vi "AlliGator All ROIs Decay Fit Non-Interactive (Fast + Individual IRF) v2.vi"(8 "error in (no error)":errorcluster, 11 "AlliGator Internal Variables DVR":refnum<data-value>) -> (0 "error out":errorcluster, 1 "Message":string, 3 "AlliGator Internal Variables DVR":refnum<data-value>)   [LabVIEW 2021, in "AlliGator Decay Fit.lvlib"]
doc: "Performs multi-ROIs NLSF decay fits for the selected ROIs.\n\nEach ROI has its own associated IRF."
uses:
  AlliGator Decay Fit.lvlib
  Internal Variables/AlliGator Internal Variables v2.ctl
  <vilib>/vision/Image Controls.llb/IMAQ Image.ctl
  Internal Variables/AlliGator Gate Image Set.ctl
  Files/AlliGator FLI Dataset Type.ctl
  Files/AlliGator Data Series Type.ctl
  Dual-Channel Datasets/AlliGator Dataset Channel.ctl
  Settings/AlliGator Gate Arithmetic.ctl
  Source Image/AlliGator Displayed Image.ctl
  Image/Named ROI Description.ctl
  Phasor Graph/AlliGator Decay Metadata v3.ctl
  Decay Preprocessing/AlliGator Decay Background Subtraction Info.ctl
  Decay Preprocessing/AlliGator Baseline Subtraction Method.ctl
  Graphs/XY Graph/XY Graph Plot Shift Parameters.ctl
  Graphs/XY Graph/XY Graph Plot Shift Method.ctl
  Decay Preprocessing/AlliGator Decay Extrapolation Parameters.ctl
  Phasor/Calibration Phasor (m, phi).ctl
  Phasor/Phasor Reference Series.ctl
  Phasor/Phasor Calibration Map v2.ctl
  Phasor/Phasor (g, s).ctl
  Phasor Graph/AlliGator Raw Phasor Plot Data v5.ctl
  Phasor/Phasor Standard Deviation Options.ctl
  Phasor Plot/AlliGator Phasor Multi-Harmonic Data.ctl
  Phasor/Phasor Harmonic Data.ctl
  Decay Fit Parameter Map/AlliGator Decay Fit Options & Parameters v3.ctl
  Fits/IRF(X)PSED/Decay Fit Options v3.ctl
  Fits/Decay Convolution/Decay Model.ctl
  Fits/Residual Type.ctl
  Fits/IRF(X)PSED/Fit Weights Type.ctl
  Fits/Non-linear Fitting Method v2.ctl
  Fits/Fit Calculation Method.ctl
  Fits/Non-linear Fitting Algorithm.ctl
  AlliGator Decay Fit Parameter Constraints 2.ctl
  Fits/IRF(X)PSED/Decay Fit Parameters In List.ctl
  Fits/IRF(X)PSED/MLE Baseline Offset Type.ctl
  Decay Preprocessing/AlliGator Decay Preprocessing Parameters.ctl
  Fits/IRF(X)PSED/Decay Fit Parameters & Derived Quantities List v2.ctl
  Fits/IRF(X)PSED/Decay Fit Result Constraint.ctl
  Decay Fit Parameter Map/AlliGator Parameter Maps Data.ctl
  Globals, Variables, Constants/AlliGator Variables List.ctl
  Settings/AlliGator Settings List.ctl
  Rich Text Box/Text Format List.ctl
  Graphs/XY Graph/XY Graph Selected Plot Info+Flag.ctl
  Graphs/XY Graph/XY Graph Refnum.ctl
  <vilib>/Utility/miscctls.llb/LVPoint32TypeDef.ctl
  Variant/Variant to Data/Variant to Boolean.vi
  Variant/Variant to Data/Variant to U16.vi
  <vilib>/Utility/error.llb/Error Cluster From Error Code.vi
  Globals, Variables, Constants/AlliGator Abort.vi
  <vilib>/ErrorRing/Error Ring.xnode
  Globals, Variables, Constants/AlliGator Globals, Variables & Constants.lvlib
  Image/Image.lvlib
  Decay Processing/AlliGator Decay Processing.lvlib
  Source Image/AlliGator Source Image.lvlib
  Strings/Strings.lvlib
  Time/Time.lvlib
  Settings/AlliGator Settings.lvlib
  Variant/Variant to Data/Variant to Data.lvlib
  GUI/GUI.lvlib
  Decay Preprocessing/AlliGator Decay Preprocessing.lvlib
  Arrays/Arrays.lvlib
  Fits/Fits.lvlib
  Notebook/Notebook.lvlib
  IRF/AlliGator IRF.lvlib
  Sound/Sound.lvlib
  Graphs/XY Graph/XY Graph Add-Ons.lvlib
  Decay Fit Parameter Map/AlliGator Decay Fit Parameter Map.lvlib
  Utilities/Utilities.lvlib
  Phasor/Phasor.lvlib
  Files/AlliGator Files.lvlib
  Internal Variables/AlliGator Internal Variables.lvlib
  Phasor Graph/AlliGator Phasor Graph.lvlib
  Phasor Plot/AlliGator Phasor Plot.lvlib
  Dual-Channel Datasets/AlliGator Dual-Channel Datasets.lvlib
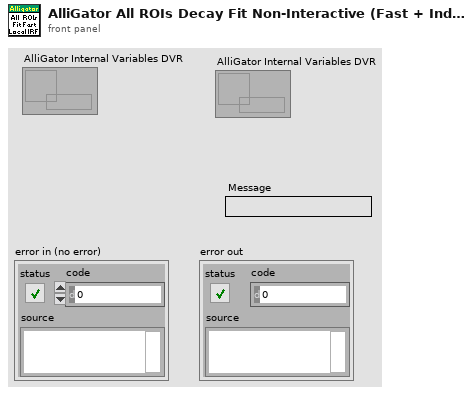
[diagram p1: front panel]
types:
  T1 = typedef "AlliGator Globals, Variables & Constants.lvlib/AlliGator Variables List.ctl" = enum16{"---- GUI ----", "GUI:Initialization Status", "GUI:State Indicators Refnum", "GUI:Original AlliGator Menu Items", "GUI:Current Action Loop State", "GUI:Script in progress", "GUI:Playback", "GUI:Loop Playback", "GUI:Search ROI Used", "GUI:Search ROI", "Decay Graph Max Legend Size", "Intensity Graph Max Legend Size", "Decay Statistics Graph Max Legend Size", "Phasor Graph Max Legend Size", "Phasor Ratio Graph Max Legend Size", "Lifetime Graph Max Legend Size", "---- Files ----", "Files:Export Dataset Frames as Individual Files", "Files:Show Batch Export Help Balloons", "Files:Frames in Dataset", "Files:ptu File Frame Start Indices", "Files:Current Frame in Dataset", "Files:Current Frame Timestamp", "Files:Dataset Loaded", "Files:Dataset Metadata", "Files:Dataset Channel", "Files:Dataset Data Description", "Files:Background Dataset Metadata", "Files:Background Dataset Channel", "Files:Background Dataset Data Description", "Files:Background File Subtraction", "Files:Background File Path", "Files:Background File Pile-up Correction", "Files:Background File Pixel Well Capacity", "Files:Background File Scaling Factor", "Files:Current Dataset Load Settings", "Files:Dataset Path", "Files:ICCD-specific Information", "Files:Macrotime Gate Separation", "------ Python Plugins ------", "Python Plugins:Information", "Python Plugins:Python Session", "Python Plugins:Valid Python Session?", "---- Source Image ----", "Source Image:ROIs", "Source Image:Current ROI", "Source Image:ROI Event Refnum", "X_Source Image:Display Range", "X_Source Image:Palette Information", "X_Source Image:Type of Displayed Image", "X_Time Gate Slider", "Source Image:Palette List", "Source Image:Scale", "Source Image:ROI Overlay Color", "Source Image:Overlay to Erase", "Source Image:Is Displayed Image Accumulated", "Source Image:White Light Image Modified", "Source Image:Mask Image Modified", "---- Image Profile Window ----", "Image Profile:Window Event Refnum", "Image Profile:IntensityType", "Image Profile:Intensity Average Type", "Image Profile:Intensity-weighted SDV", "Image Profile:Box Profile Type", "Image Profile:Window Open", "Image Profile:Plotted Fit Parameter", "------ Phasor Graph -------", "Phasor Graph:Show Line", "---- Phasor Plot ---", "Phasor Plot:Parameters Changed", "Phasor Plot:FLI Dataset Modified since last Calculation", "Phasor Harmonics Data", "Selected Phasor Harmonics", "Phasor Harmonic Manager Event Refnum", "Phasor Plot:ROIs", "Phasor Plot:Current ROI", "Phasor Plot:ROI Event Refnum", "Phasor Plot:Image Reference Points", "Phasor Plot:Computed", "Phasor Plot:Palette Information", "Phasor Plot:Palette List", "Phasor Plot:Phasor Ratio Palette Information", "Phasor Plot:Phasor Ratio Palette List", "Phasor Plot:Image Scale", "Phasor Plot:Image Overlay to Erase", "Phasor Plot:Image Elements to Update", "Phasor Plot:Current Calculation Parameters", "Phasor Plot:Current Calibration Options", "Phasor Plot:Reset Cumulated Phasor Plot", "Phasor Plot:Reference 1", "Phasor Plot:Lifetime Reference 1", "Phasor Plot:Reference 1 Frequency", "Phasor Plot:Reference 2", "Phasor Plot:Lifetime Reference 2", "Phasor Plot:Reference 2 Frequency", "---- Decay Analysis ----", "Number of Selected Decays to Fit", "LS Fit Results", "LAR Fit Results", "BS Fit Results", "Last Decay Max - Min", "Best Fit Parameters", "Best Fit Parameter Names", "Actual Size X", "Actual Size Y", "Binning X", "Binning Y", "Actual # Gates", "Dataset Number", "Gates to...", "Gates Skipped", "Gates to keep", "Gate Step", "Gate Separation", "Reversed Gates", "Pile-up Correction", "Pixel Well Capacity", "Background Subtracted", "Background Subtraction Method", "Background Definition Range", "Background File (deprecated)", "Number of Dataset Accumulated", "Array of Accumulated Dataset Paths", "Do Averaged Datasets", "Destination File Path", "Process Plot Target", "Use 1/D as Phasor Frequency", "---- Decay Fit Parameter Map -----", "Decay Fit Parameter Map:Palette Information", "Decay Fit Parameter Map:Palette List", "Decay Fit Parameter Map:X Resolution", "Decay Fit Parameter Map:Y Resolution", "Decay Fit Parameter Map:Use Decay Fit Result Constraints", "Decay Fit Parameter Map:Decay Fit Result Constraints", "Decay Fit Parameter Map:Decay Fit Result Constraints Applied", "---- Parameter Map ----", "Parameter Map:Palette Information", "Parameter Map:Palette List", "------- Local Decay Window ---------", "Local Decay Graph Window:Event Refnum", "Local Decay Graph Window:Use normalized IRF for convolution", "----- Miscellaneous ----", "Misc:Skippable Dialog Windows Status"}
  T2 = typedef "IMAQ Image.ctl" = refnum<image>
  T3 = typedef "AlliGator Settings.lvlib/AlliGator Settings List.ctl" = enum16{"GUI:Visible Settings Tab", "GUI:Last Run Version", "Source Image:Use Image Histogram for Contrast", "Source Image:Low Count Pixels Rejection Options", "Source Image:High Count Pixels Rejection Options", "Source Image:Use Image Brightness", "Source Image:Blend Overlay with Image Background", "Source Image:Use Fixed ROI Diameter", "Source Image:ROI Diameter", "Source Image:ROI Center Color", "Source Image:Peak Threshold", "Source Image:Intensity Threshold", "Source Image:Image Binning Options", "Source Image:Image Smoothing Options", "Source Image:Image Histogram Active", "Source Image:Invert Binary Mask", "Source Image:Hot Pixel Removal", "Source Image:Overlay Analyzed ROI Center", "Source Image:Auto-Adjust Contrast", "Source Image:Histogram Lower Percentile", "Source Image:Histogram Upper Percentile", "Source Image:Save Source Image", "Source Image:Scale Bar Options", "Source Image:Image Resolution (Pixel Size)", "Source Image:Flatfield Correction", "Source Image:Show Dead Left Columns Correction", "Source Image:Dead Left Columns Correction", "Source Image:Image Pre-Processing Operations Order", "Source Image:Overlay ROI Median", "Source Image:Median Overlay Color", "Data Information:Gate Width", "Data Information:Nanotime Gate Separation", "Data Information:Macrotime Gate Separation", "Data Information:Gate Step", "Data Information:# Gates", "Data Information:Gate Image Exposure", "Data Information:Gate Image Integration", "Data Information:Gates to Skip", "Data Information:Gates to Keep", "Data Information:Define Gates to", "Data Information:Channel Name", "Data Information:Available Channel Names", "Data Information:Channel Arithmetic", "Data Information:Background File Subtraction", "Data Information:Background File", "Data Information:Background Scaling Factor", "Data Information:Background Pile-up Correction", "Data Information:Background Pixel Well Capacity", "Data Information:Laser Period", "Data Information:SYNC Period", "Data Information:Pile-up Correction", "Data Information:Pixel Well Capacity", "Data Information:Dataset Scaling Factor", "Fluorescence Decay_Decay Pre-Processing:Reverse Gates", "Fluorescence Decay_Decay Pre-Processing:Verbose Decay Pre-Processing", "Fluorescence Decay_Decay Pre-Processing:Use Decay Pre-Processing", "Fluorescence Decay_Decay Pre-Processing:Background Subtraction", "Fluorescence Decay_Decay Pre-Processing:Background Definition Range", "Fluorescence Decay_Decay Pre-Processing:Baseline Subtraction Method", "Fluorescence Decay_Decay Pre-Processing:Decay Pre-Processing Operations Order", "Fluorescence Decay_Decay Pre-Processing:Smoothing Parameter", "Fluorescence Decay_Decay Pre-Processing:Shift Decay", "Fluorescence Decay_Decay Pre-Processing:Decay Shift Parameters", "Fluorescence Decay_Decay Pre-Processing:Fold Decay", "Fluorescence Decay_Decay Pre-Processing:# Folds", "Fluorescence Decay_Decay Pre-Processing:1-Normalize Decay", "Fluorescence Decay_Decay Pre-Processing:[0-1]-Normalize Decay", "Fluorescence Decay_Decay Pre-Processing:Smoothen Decay", "Fluorescence Decay_Decay Pre-Processing:Extrapolate Decay", "Fluorescence Decay_Decay Pre-Processing:Use Periodicity", "Fluorescence Decay_Decay Pre-Processing:Use Cursors", "Fluorescence Decay_Decay Pre-Processing:Tail Fraction", "Fluorescence Decay_Decay Pre-Processing:Head Fraction", "Fluorescence Decay_Decay Pre-Processing:Additional Points", "Fluorescence Decay_Decay Pre-Processing:Straighten Decay", "Fluorescence Decay_Decay Pre-Processing:Constant Background", "Fluorescence Decay_Decay Pre-Processing:Pixel-Normalize Decay", "Fluorescence Decay_Advanced Analysis:Extract IRF instead of Decay", "Fluorescence Decay_Advanced Analysis:IRF Extraction Options", "Fluorescence Decay_Advanced Analysis:IRF Optimization Options", "Fluorescence Decay_Advanced Analysis:Square Pulse Options", "Fluorescence Decay_Advanced Analysis:IRF Order", "Fluorescence Decay_Advanced Analysis:IRF Time Constants", "Fluorescence Decay_Advanced Analysis:Wavelet Analysis Options", "Fluorescence Decay_Advanced Analysis:Average Lifetime Options", "Fluorescence Decay_Fit Options:Fit Options", "Fluorescence Decay_Fit Options:Use Legacy Fitting Approach", "Fluorescence Decay_Fit Options:Use Data Information Laser Period", "Fluorescence Decay_Fit Parameters:Displayed Fit Parameters", "Fluorescence Decay_Fit Parameters:Fit Parameter Constraints", "Fluorescence Decay_Fit Parameters:Export Tabulated Results", "Fluorescence Decay_Fit Parameters:MLE Baseline Offset Type", "Fluorescence Decay_Fit Parameters:MLE Baseline Offset", "Fluorescence Decay_Fit Parameters:Guess Parameter Names", "Fluorescence Decay_Fit Parameters:Guess Parameter Values", "Fluorescence Decay_Fit Parameters:Guess Parameters Options", "Fluorescence Decay_Fit Parameters:Optimal Offset Selection Criterion", "Fluorescence Decay_Styles:Show Last Decay Only", "Fluorescence Decay_Styles:Decay Graph Color Array", "Fluorescence Decay:Decay Graph Active", "Fluorescence Decay Statistics:Min Peak Value", "Fluorescence Decay Statistics:Reject Low Decay Peak Pixels", "Fluorescence Decay Statistics:Reject High Decay Peak Pixels", "Fluorescence Decay Statistics:Max Peak Value", "Time Traces:Use File Timestamp", "Time Traces:Time Step", "Time Traces:Use Intensity Correction File", "Time Traces:Intensity Correction File", "Phasor Plot:Phasor Plot Smoothing Options", "Phasor Plot:Phasor Plot Size", "Phasor Plot:Phasor Plot Graphics Options", "Phasor Plot:Cumulative Phasor Plot", "Phasor Plot:Use Phasor Brightness", "Phasor Plot:Blend Overlay with Phasor Background", "Phasor Plot:Save Phasor Plot", "Phasor Plot:Show References", "Phasor Plot:Phasor Ratio Decay Range", "Phasor Plot:Exponential Fading", "Phasor Plot:Phasor Ratio Reference Colors", "Phasor Plot:Reference Radius", "Phasor Plot:Show Color Map Vertices", "Phasor Plot:Phasor Plot Active", "Phasor Plot:Phasor Ratio Color Map Type", "Phasor Plot:Phasor Ratio Color Map", "Phasor Plot:Phasor Ratio Display Range", "Phasor Plot:Selected Image ROI(s)", "Phasor Plot:All Image ROIs", "Phasor Plot:Selected Phasor Plot ROI(s)", "Phasor Plot:All Phasor Plot ROIs", "Phasor Plot:Phasor Ratio Color-Coded Quantity", "Phasor Plot:Store Phasor Harmonics", "Phasor Plot:Draw Reference Segment", "Phasor Plot:User-Defined Quantity", "Phasor Plot:Color Scale High Color", "Phasor Plot:Color Scale Low Color", "Phasor Plot:Intensity-weighted Phasor Plot", "Phasor Graph:Phasor Frequency", "Phasor Graph:Phasor Ratio Type", "Phasor Graph:Pixel-level Phasor Computation", "Phasor Graph:Save Phasor Graph", "Phasor Graph:Phasor Graph Active", "Phasor Graph:Phasor SDV Options", "Phasor Graph:Intensity-weighted Phasor Graph", "Phasor Graph:Define Shortest Lifetime as", "Phasor Calibration:Use Backup Calibration if needed", "Phasor Calibration:Backup Calibration Type", "Phasor Calibration:Calibration Type", "Phasor Calibration:Calibration Lifetime", "Phasor Calibration:Calibration Map Algorithm", "Single-Exponential Phasor Locus (SEPL):Gate Parameters", "Single-Exponential Phasor Locus (SEPL):User-defined Gate", "Single-Exponential Phasor Locus (SEPL):User-defined IRF", "Single-Exponential Phasor Locus (SEPL):Phasor Parameters", "Single-Exponential Phasor Locus (SEPL):Decay & IRF Parameters", "Single-Exponential Phasor Locus (SEPL):Display Parameters", "Lifetime Analysis:Decay Analysis Parameters", "Lifetime Analysis:Lifetime Map Active", "Plugins:Python Settings", "Miscellaneous:Verbose Mode", "Miscellaneous:Beep after Script", "Miscellaneous:Saved Image File Format", "Miscellaneous:Exported Gate Image Settings", "Miscellaneous:Include Loading in Timing", "Miscellaneous:Verbose Settings Mode", "Miscellaneous:Histogram Options", "Miscellaneous:Beep on Error", "Miscellaneous:# Logical Processors Used", "Miscellaneous:ROI Description Max Characters", "Miscellaneous:Verbose Error Mode", "Miscellaneous:Transparent Mask Color"}
  T4 = typedef "Image.lvlib/Named ROI Description.ctl" = cluster{"ROI Descriptor":T5, "ROI Name":string, "Overlay Color":u32}
  T5 = typedef "ROI Descriptor" = cluster{"Global Rectangle":i32[], "Contours":cluster{"ID":enum32{"External", "Internal"}, "Type":u32, "Coordinates":i32[]}[]}
  T6 = typedef "Notebook.lvlib/Text Format List.ctl" = enum16{"Message", "Result", "Error", "Setting", "Verbose", "Warning"}
  T7 = typedef "AlliGator Internal Variables.lvlib/AlliGator Internal Variables v2.ctl" = cluster{"----------------------------- Images -----------------------------":u8, "Displayed Image":T2, "White Light Image":T2, "Mask Image":T2, "ROI Mask Image":T2, "Current Dataset Images 1":T8, "Background Dataset Images 1":T8, "Current Dataset Images 2":T8, "Background Dataset Images 2":T8, "Current Dataset Arithmetic Images":T8, "Accumulated Dataset Images 1":T8, "Accumulated Dataset Images 2":T8, "Accumulated Dataset Arithmetic Images":T8, "----------------------------- File Paths -----------------------------":u8, "Phasor Plot Image":T2, "Decay Fit Parameter Map Image":T2, "Parameter Map Image":T2, "Single Data Point Path":path, "White Light Image Path":path, "Mask Image Path":path, "Time-Series Folder":path, "[Time-Series Paths]":path[], "----------------------------- FLI Dataset -----------------------------":u8, "Current Dataset":i32, "Single Dataset Type":T9, "Current Folder":string, "AlliGator Data Series Type":T10, "# Datasets":i32, "Dual-Channel Dataset":bool, "Selected Channel Name":string, "Dataset Channel":T11, "Channel Arithmetic":T12, "Dual-Channel Background Dataset":bool, "Background Channel":T11, "Dual-Channel Accumulated Dataset":bool, "Start Time":dbl, "[Time-Series Timestamps]":dbl[], "[Intensity Corrections]":dbl[], "Time Series Script":bool, "Type of Displayed Image":T13, "Gate Image Slide":u16, "# Gates":i32, "ROIs":T4[], "----------------------------- Decays -----------------------------":u8, "ROI Decay":cluster{"t Array":dbl[], "I Array":dbl[]}, "Valid Decay":bool, "Decay  Metadata":T14, "Reference Decay Plot Name":string, "Reference Decay":cluster{"t Array":dbl[], "I Array":dbl[]}, "Decay Shift Plot":cluster{"Time Stamps":dbl[], "Decay Shifts":dbl[]}, "[Decays Max Values]":sgl[], "[Decays Min Values]":sgl[], "----------------------------- Calibration -----------------------------":u8, "Calibration Phasor":T20, "Calibration Phasor Series":T21, "Phasor Calibration Map":T22, "Calibration Map MD5 Digest":string, "----------------------------- Phasor Graph -----------------------------":u8, "Last Raw Phasor":T23, "Last Calibrated Phasor":T23, "Last Calibrated Phasor SDV":T23, "Phasor Graph:Phasor Plot":cluster{"g Array":dbl[], "s Array":dbl[]}, "Phasor Graph:Phasor SDV Plot":cluster{"g Array":dbl[], "s Array":dbl[]}, "[Phasor Graph:Raw Phasor Plots]":T24[], "Phasor Plot locked to Ref 1":i32, "[Phasor Plot(s) locked to Ref 1]":i32[], "[Phasor Plot(s) locked to Ref 2]":i32[], "[Pixel Phasors]":T23[], "----------------------------- Phasor Plot -----------------------------":u8, "[[Sum Image]]":dbl[][], "[[CSG Phasors]]":csg[][], "[[Valid Pixel?]]":bool[][], "[[Phasor Ratios]]":dbl[][], "[[Average Lifetimes]]":dbl[][], "Amplitude Weighted Average Lifetime":bool, "I/m/phi Dataset":cluster{"I/m/phi Dataset?":bool, "Base Frequency":dbl[unit], "Harmonic Orders":u8[]}, "Multi Phasor Plot Data":T26, "----------------------------- Decay Fit Parameter Map -----------------------------":u8, "Decay Fit Options & Parameters":T28, "Fit Options: Decay Preprocessing Parameters":T39, "Fit Options: Reference Decay":cluster{"t Array":dbl[], "I Array":dbl[]}, "Is Full Image Parameters Map":bool, "Is Single-Pixels Parameters Map":bool, "NLSF Parameters Map X Resolution":i32, "NLSF Parameters Map Y Resolution":i32, "[Single Decay Fit Parameters]":dbl[], "Fit Model":T30, "[[Multiple Decays Fit Parameters]]":dbl[][], "[[Multiple Decays Fit Parameter SDVs]]":dbl[][], "[[IRFs]]":dbl[][], "[ROI Descriptors]":T5[], "IRF Array Time Axis":dbl[], "Decay Array Time Axis":dbl[], "[Decay Fit Parameter Names]":T40[], "[Decay Sum]":dbl[], "Array of Decay Fit Result Constraints":T41[], "Selected ROIs Array":bool[], "----------------------------- Parameter Maps -----------------------------":u8, "[Map Set Names]":string[], "[Parameter Maps]":T42[], "[[User-defined Quantities]]":dbl[][], "User-defined Quantity":string}
  T8 = typedef "AlliGator Internal Variables.lvlib/AlliGator Gate Image Set.ctl" = cluster{"SGL Image Max":T2, "SGL Image Sum":T2, "SGL Gate Images":T2[], "SGL Image Min":T2}
  T9 = typedef "AlliGator Files.lvlib/AlliGator FLI Dataset Type.ctl" = enum16{"HDF5 FLI Dataset", "Gate Image Folder", ".sdt FLI Dataset (Becker & Hickl)", ".ptu FLI Dataset (PicoQuant)", "SS1 FLI Dataset", "SS2 FLI Dataset", "I/m/phi Dataset", ".bin FLI Dataset (PicoQuant Binned)", ".bin FLI Dataset (Piccolo Binned)", ".mat FLI Dataset"}
  T10 = typedef "AlliGator Files.lvlib/AlliGator Data Series Type.ctl" = enum16{"Not a Supported Series", "Gate Images Folder Series", "SwissSPAD 2 Dataset Series", "B&H FLI Dataset Series", "PicoQuant PTU FLI Dataset Series", "PicoQuant BIN FLI Dataset Series", "Piccolo hist BIN FLI Dataset Series", "HDF5 FLI Dataset Series"}
  T11 = typedef "AlliGator Dual-Channel Datasets.lvlib/AlliGator Dataset Channel.ctl" = enum16{"G2", "INT"}
  T12 = typedef "AlliGator Settings.lvlib/AlliGator Gate Arithmetic.ctl" = enum16{"None", "INT-G2", "G2/INT*<INT>", "(1 - G2/INT)*<INT>"}
  T13 = typedef "AlliGator Source Image.lvlib/AlliGator Displayed Image.ctl" = enum16{"Single Gate", "Sum of All Gates", "Max of All Gates", "Min of All Gates", "-", "White Ligth Image", "Mask Image"}
  T14 = typedef "AlliGator Phasor Graph.lvlib/AlliGator Decay Metadata v3.ctl" = cluster{"ROI Descriptor":T5, "ROI Center":cluster{"X":i32, "Y":i32}, "Decay Background Subtraction Info":T15, "Decay Reverted":bool, "Decay Smoothened":bool, "Decay Straightened":bool, "Fitted Tau (Decay Straightening)":dbl, "Decay Shift Parameters":T17, "Decay Shifted":bool, "Decay Extrapolated":bool, "Decay Extrapolation Parameters":T19, "Decay Normalized":bool, "Fold Decay":bool, "# Folds":u32}
  T15 = typedef "AlliGator Decay Preprocessing.lvlib/AlliGator Decay Background Subtraction Info.ctl" = cluster{"Laser Period":dbl[unit], "Gate Duration":dbl[unit], "Baseline Subtraction Method":T16, "Background Definition Range":cluster{"Min Gate":dbl[unit], "Max Gate":dbl[unit]}, "Total Intensity w/o Bkgd Subtraction":dbl, "Bkgd-subtracted Intensity (exp)":dbl, "# Data Points":i32, "Background/Gate":dbl, "Fitted Lifetime":dbl[unit], "Bkgd-subtracted Intensity (theo)":dbl}
  T16 = typedef "AlliGator Decay Preprocessing.lvlib/AlliGator Baseline Subtraction Method.ctl" = enum16{"Mean", "Min", "Square Gated Single-Exponential", "File", "Constant"}
  T17 = typedef "XY Graph Add-Ons.lvlib/XY Graph Plot Shift Parameters.ctl" = cluster{"Type":T18, "Shift":dbl[unit], "Threshold":dbl, "Rotate":bool}
  T18 = typedef "XY Graph Add-Ons.lvlib/XY Graph Plot Shift Method.ctl" = enum16{"Default", "CFD", "Threshold", "Cross-Correlation"}
  T19 = typedef "AlliGator Decay Preprocessing.lvlib/AlliGator Decay Extrapolation Parameters.ctl" = cluster{"Additional Points":u32, "Head Fraction":dbl, "Fitted Tau":dbl, "Use Periodicity":bool, "Use Cursors":bool, "Tail Fraction":dbl}
  T20 = typedef "Phasor.lvlib/Calibration Phasor (m, phi).ctl" = cluster{"m":dbl, "phi":dbl, "Phasor Frequency":dbl[unit], "Reference Lifetime":dbl[unit]}
  T21 = typedef "Phasor.lvlib/Phasor Reference Series.ctl" = cluster{"m Array":dbl[], "phi Array":dbl[], "Phasor Frequency":dbl[unit], "Calibration Lifetime":dbl[unit]}
  T22 = typedef "Phasor.lvlib/Phasor Calibration Map v2.ctl" = cluster{"Phasor Frequency":dbl[unit], "Calibration Lifetime":dbl[unit], "ROI Centers":cluster{"X":i32, "Y":i32}[], "ROI Descriptors":T5[], "Map Resolution X":i32, "Map Resolution Y":i32, "z Array":cdb[]}
  T23 = typedef "Phasor.lvlib/Phasor (g, s).ctl" = cluster{"g":dbl, "s":dbl}
  T24 = typedef "AlliGator Phasor Graph.lvlib/AlliGator Raw Phasor Plot Data v5.ctl" = cluster{"Phasor Plot Name":string, "Raw Phasor Plot":T23[], "Phasor Frequency":dbl[unit], "[Decay Metadata]":T14[], "Raw Phasor Plot SDV":T23[], "Phasor SDV Options":T25, "[Calibration Phasor]":T20[], "Intensity Array":dbl[]}
  T25 = typedef "Phasor.lvlib/Phasor Standard Deviation Options.ctl" = cluster{"Compute Estimated SDV":bool, "# Replicas":u32, "Use Estimated Average Phasor":bool}
  T26 = typedef "AlliGator Phasor Plot.lvlib/AlliGator Phasor Multi-Harmonic Data.ctl" = cluster{"Base Frequency":dbl[unit], "# Harmonics":u8, "Harmonic Orders":u8[], "Phasor Plot Settings Checksum":u64, "Phasor Harmonic Data Array":T27[]}
  T27 = typedef "Phasor.lvlib/Phasor Harmonic Data.ctl" = cluster{"Phasor Harmonic Name":string, "Phasor Plot Settings Checksum":u64, "Phasor Frequency":dbl[unit], "Base Frequency":dbl[unit], "Harmonic Order":u8, "Phasor Plot Parameters":string, "Phasor Array [[CSG]]":csg[][], "Dataset File Path":path}
  T28 = typedef "AlliGator Decay Fit Parameter Map.lvlib/AlliGator Decay Fit Options & Parameters v3.ctl" = cluster{"SYNC Period":dbl[unit], "Fit Options":T29, "Fit Parameter Constraints":T36[], "MLE Baseline Offset":dbl, "MLE Baseline Offset Type":T38}
  T29 = typedef "Fits.lvlib/Decay Fit Options v3.ctl" = cluster{"Show Fit Residuals":bool, "Fit Model":T30, "Residual Type":T31, "Max Decay Percentile":dbl, "Min Decay Percentile":dbl, "Show Full Decay":bool, "Weights":T32, "Fitting Method":T33, "Compute Parameter Uncertainties":bool, "Periodic Boundaries":bool, "Model Calculation":T34, "Period":dbl[unit], "Termination Criteria":cluster{"Max Iterations":i32, "Max Function Calls":i32, "Max Time":dbl[unit], "Function Tolerance":dbl, "Parameter Tolerance":dbl, "Gradient Tolerance":dbl, "Min Lambda":dbl, "Max Lambda":dbl, "Initial Tick Count":u32}, "Offset Resolution":dbl[unit], "Use Local IRF":bool, "Fitting Algorithm":T35, "Show Confidence Interval ":bool, "Confidence Level":dbl}
  T30 = typedef "Fits.lvlib/Decay Model.ctl" = enum16{"1-Exponential", "2-Exponentials"}
  T31 = typedef "Fits.lvlib/Residual Type.ctl" = enum16{"Standard", "Normalized", "Reduced"}
  T32 = typedef "Fits.lvlib/Fit Weights Type.ctl" = enum16{"Unweighted", "1/Variance", "Best of All"}
  T33 = typedef "Fits.lvlib/Non-linear Fitting Method v2.ctl" = enum16{"Least Square", "Least Absolute Residual", "Bisquare", "MLE", "-", "Best of All"}
  T34 = typedef "Fits.lvlib/Fit Calculation Method.ctl" = enum16{"Simulation", "Convolution", "Integration"}
  T35 = typedef "Fits.lvlib/Non-linear Fitting Algorithm.ctl" = enum16{"Levenberg-Marquardt", "Trust-Region Dogleg"}
  T36 = typedef "AlliGator Decay Fit.lvlib/AlliGator Decay Fit Parameter Constraints 2.ctl" = cluster{"Fit Parameter":T37, "Min Value":dbl, "Max Value":dbl, "Global":bool, "Used":bool}
  T37 = typedef "Fits.lvlib/Decay Fit Parameters In List.ctl" = enum16{"Offset", "Baseline", "A_1", "tau_1", "A_2", "tau_2"}
  T38 = typedef "Fits.lvlib/MLE Baseline Offset Type.ctl" = enum32{"Absolute", "Percentage"}
  T39 = typedef "AlliGator Decay Preprocessing.lvlib/AlliGator Decay Preprocessing Parameters.ctl" = cluster{"Background Subtraction":bool, "Straighten Decay":bool, "Reverse Gates":bool, "1-Normalized Decay":bool, "Smoothen Decay":bool, "Smoothing Parameter":dbl, "Shift Decay":bool, "Decay Shift Parameters":T17, "Extrapolate Decay":bool, "Additional Points":u32, "Head Fraction":dbl, "Pixel-Normalize Decay":bool, "Use Periodicity":bool, "Use Cursors":bool, "Tail Fraction":dbl, "Use Decay Pre-Processing":bool, "Fold Decay":bool, "# Folds":u32, "[0-1]-Normalized Decay":bool}
  T40 = typedef "Fits.lvlib/Decay Fit Parameters & Derived Quantities List v2.ctl" = enum16{"Offset", "Baseline", "A_1", "tau_1", "A_2", "tau_2", "<tau>_a", "f1_a", "f2_a", "<tau>_i", "f1_i", "f2_i", "-", "R^2", "Chi^2"}
  T41 = typedef "Fits.lvlib/Decay Fit Result Constraint.ctl" = cluster{"Fit Parameter":enum16{"Offset", "Baseline", "A_1", "tau_1", "A_2", "tau_2", "<tau>_a", "f1_a", "f2_a", "<tau>_i", "f1_i", "f2_i", "-", "R^2", "Chi^2", "Max Relative Residual", "<Residual ACF>", "Residual ACF SDV", "tau_2/tau_1"}, "Min Value":dbl, "Max Value":dbl, "Use Constraint":bool}
  T42 = typedef "AlliGator Decay Fit Parameter Map.lvlib/AlliGator Parameter Maps Data.ctl" = cluster{"Map Set Name":string, "[Parameter Names]":string[], "[[Parameters]]":dbl[][], "[[Parameter SDVs]]":dbl[][], "Decay Array Time Axis":dbl[], "[[IRFs]]":dbl[][], "IRF Array Time Axis":dbl[], "X Resolution":i32, "Y Resolution":i32, "Intensity Array":dbl[]}
  T43 = typedef "AlliGator Settings.lvlib/AlliGator Pixel Counts Constraints.ctl" = cluster{"High Count Pixels Rejection Options":T44, "Low Count Pixels Rejection Options":T45}
  T44 = typedef "AlliGator Settings.lvlib/AlliGator High Count Pixels Rejection Options.ctl" = cluster{"Background High Threshold Factor":dbl, "Fixed High Background Threshold":dbl, "Reject High Count Pixels":bool, "High Percentile":dbl}
  T45 = typedef "AlliGator Settings.lvlib/AlliGator Low Count Pixels Rejection Options.ctl" = cluster{"Background Low Threshold Factor":dbl, "Fixed Low Background Threshold":dbl, "Reject Low Count Pixels":bool, "Low Percentile":dbl}
  T46 = cluster{"Decay Peak Constraint":bool, "Min":dbl, "Max":dbl}
  T47 = typedef "XY Graph Add-Ons.lvlib/XY Graph Selected Plot Info+Flag.ctl" = cluster{"Multiplot XY Graph":T48, "Mouse Coordinates":T49, "Plot Index":i32, "Flag":bool}
  T48 = typedef "XY Graph Add-Ons.lvlib/XY Graph Refnum.ctl" = refnum<vi>
  T49 = typedef "LVPoint32TypeDef.ctl" = cluster{"Horizontal":i32, "Vertical":i32}
  T50 = cluster{"t Axis":dbl[], "ROI Intensity Array":dbl[]}
  T51 = cluster{"IRF Array Time Axis":dbl[], "[IRF Values]":dbl[]}
  T52 = typedef "Rich Text Box.lvlib/Text Formatting.ctl" = cluster{"Font":string, "Text Color":T53, "Background Color":T53, "Style":T54, "Font Size":dbl, "Alignment":T55}
  T53 = typedef "Rich Text Box.lvlib/Text Colors.ctl" = enum16{"Unchanged", "Black", "Blue", "Cyan", "Maroon", "Gray", "Violet", "Green", "Light Green", "Orange", "Yellow", "Magenta", "Red", "White"}
  T54 = typedef "Rich Text Box.lvlib/Text Style.ctl" = enum16{"Regular", "Bold", "Italic", "Underline", "Strikeout"}
  T55 = typedef "Rich Text Box.lvlib/Text Alignment.ctl" = enum16{"Left", "Right", "Center"}
  T56 = typedef "AlliGator Decay Fit.lvlib/AlliGator Decay Fit Output Options.ctl" = cluster{"Fit Model":T30, "Decay Fit Parameter Array":T40[]}
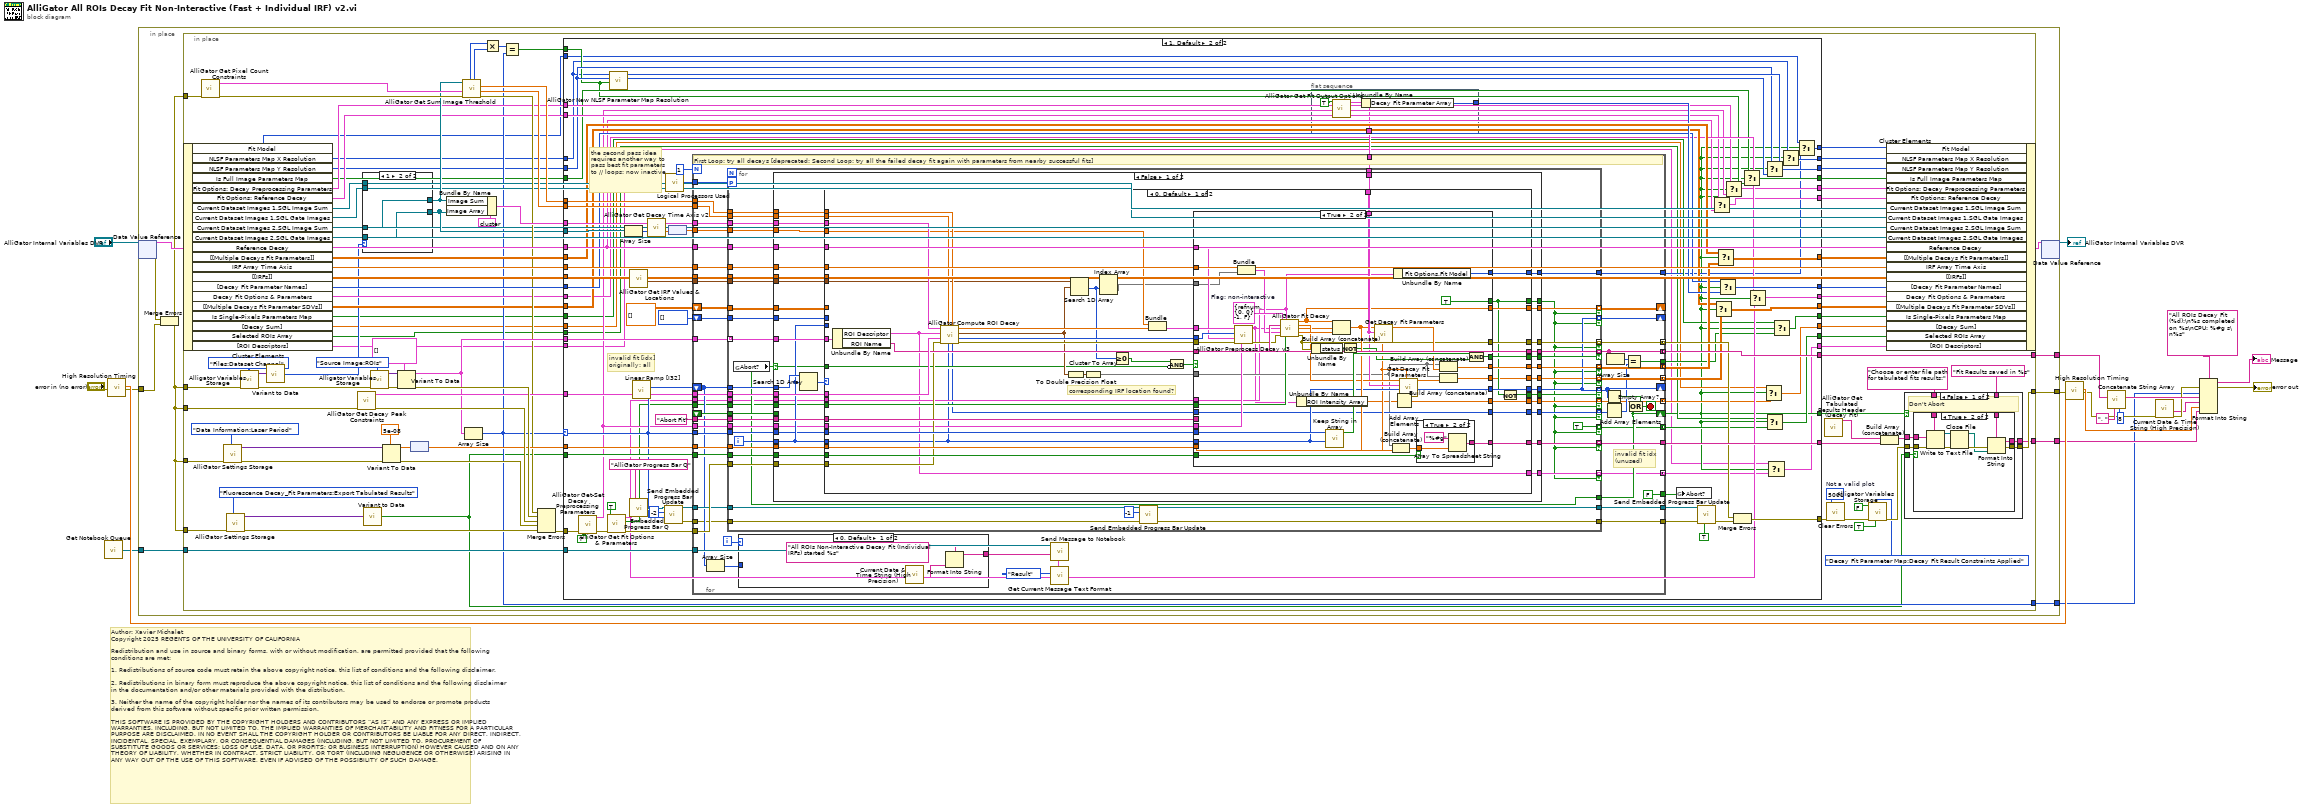
[diagram p0: block diagram]
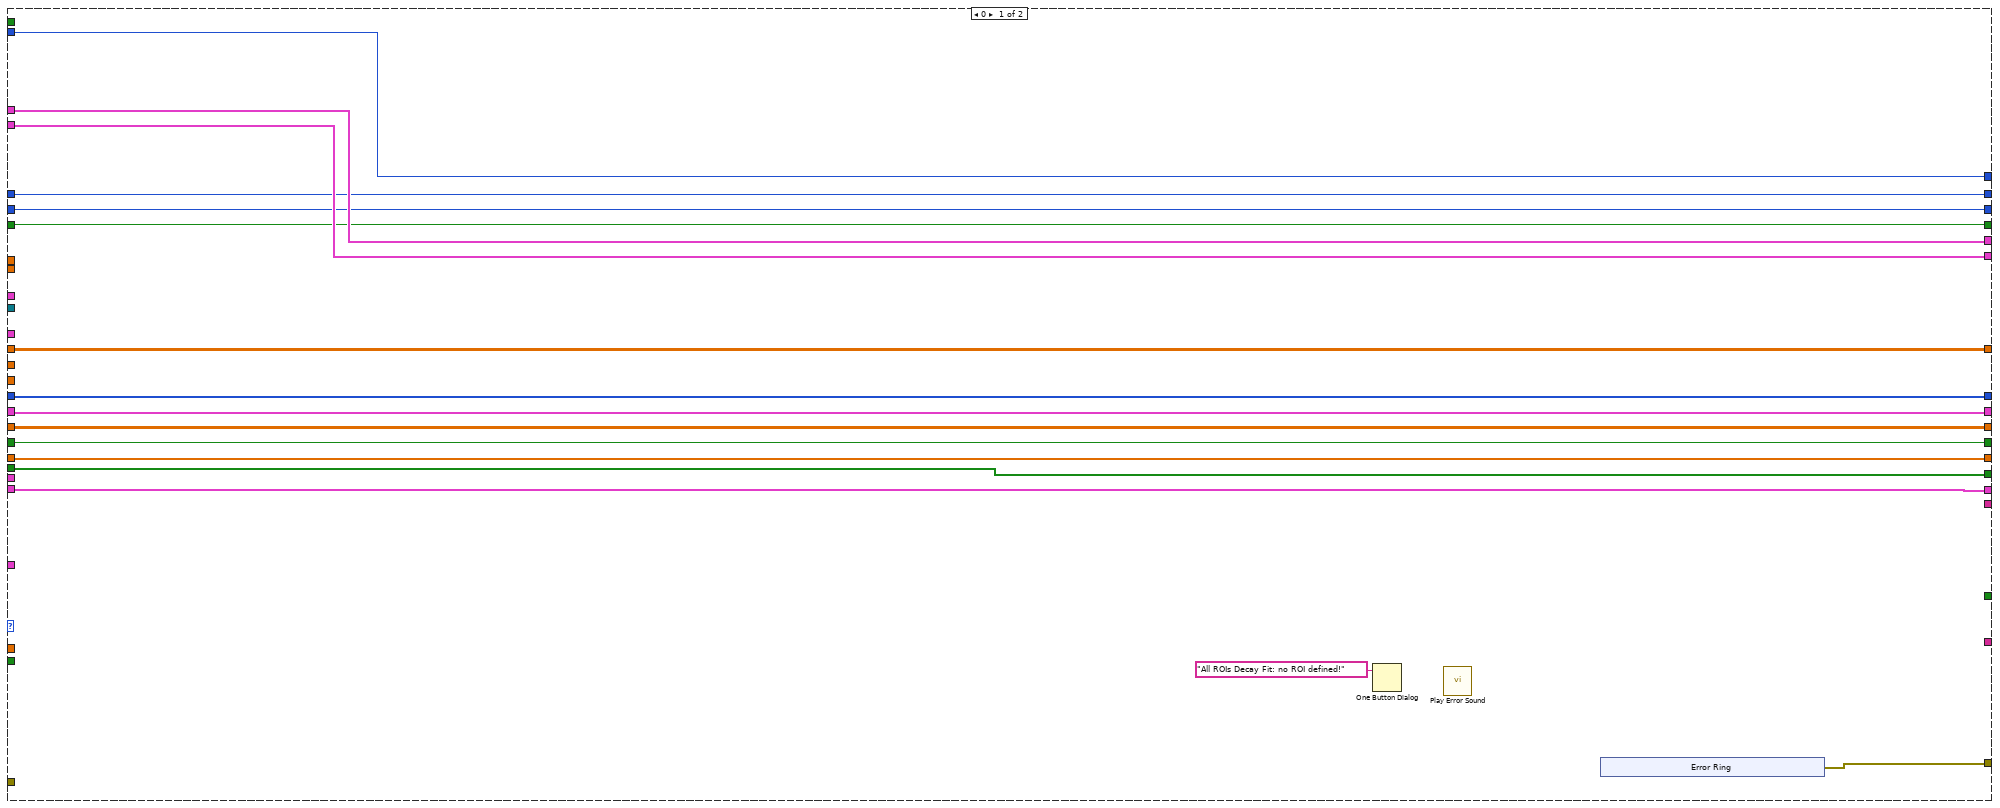
[diagram p3: hidden frame]
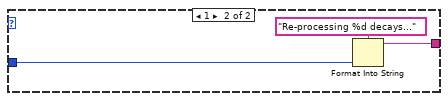
[diagram p4: hidden frame]
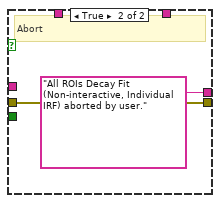
[diagram p10: hidden frame]
diagram:
  # "Author: Xavier Michalet\nCopyright 2025 REGENTS OF THE UNIVERSITY OF CALIFORNIA\n\nRedistribution and use in source and binary forms, with or without modification, are permitted provided that the following conditions are met:\n\n1. Redistributions of source code must retain the above copyright notice, this list of conditions and the following disclaimer.\n\n2. Redistributions in binary form must reproduce the above copyright notice, this list of conditions and the following disclaimer in the documentation and/or other materials provided with the distribution.\n\n3. Neither the name of the copyright holder nor the names of its contributors may be used to endorse or promote products derived from this software without specific prior written permission.\n\nTHIS SOFTWARE IS PROVIDED BY THE COPYRIGHT HOLDERS AND CONTRIBUTORS “AS IS” AND ANY EXPRESS OR IMPLIED WARRANTIES, INCLUDING, BUT NOT LIMITED TO, THE IMPLIED WARRANTIES OF MERCHANTABILITY AND FITNESS FOR A PARTICULAR PURPOSE ARE DISCLAIMED. IN NO EVENT SHALL THE COPYRIGHT HOLDER OR CONTRIBUTORS BE LIABLE FOR ANY DIRECT, INDIRECT, INCIDENTAL, SPECIAL, EXEMPLARY, OR CONSEQUENTIAL DAMAGES (INCLUDING, BUT NOT LIMITED TO, PROCUREMENT OF SUBSTITUTE GOODS OR SERVICES; LOSS OF USE, DATA, OR PROFITS; OR BUSINESS INTERRUPTION) HOWEVER CAUSED AND ON ANY THEORY OF LIABILITY, WHETHER IN CONTRACT, STRICT LIABILITY, OR TORT (INCLUDING NEGLIGENCE OR OTHERWISE) ARISING IN ANY WAY OUT OF THE USE OF THIS SOFTWARE, EVEN IF ADVISED OF THE POSSIBILITY OF SUCH DAMAGE."
  n1 = call "Get Notebook Queue.vi"() -> ("Notebook Queue"=w2:refnum<queue>)  [unwired: 9 in]
  n2 = call "High Resolution Timing.vi"("Error In"="error in (no error)") -> ("elapsed (relative) seconds"=w14:dbl, "Error Out"=w10:errorcluster)  [unwired: 16 in, 1 out]
  n3 = in-place {
    in-place-border: [w28] -> w9
    in-place-border: [w27] -> w11
    in-place-border: w10 -> [w24]
    in-place-border: [w25] -> w8
    in-place-border: [w23] -> w5
    in-place-border: w2 -> [w22]
    n4 = in-place-dvr #1("AlliGator Internal Variables DVR") -> (w30:T7, w26:errorcluster)
    n5 = Merge Errors(w26, w24) -> (w21:errorcluster)
    n6 = in-place {
      in-place-border: [w105] -> w28
      in-place-border: [w112] -> w27
      in-place-border: [w100] -> w25
      in-place-border: [w55] -> w23
      in-place-border: w22 -> [w79]
      in-place-border: w21 -> [w70]
      in-place-border: w21 -> [w66]
      in-place-border: w21 -> [w67]
      in-place-border: w21 -> [w68]
      in-place-border: w21 -> [w69]
      w82 = 5001  # Not a valid plot
      n7 = in-place-cluster #2(w30) -> ("Fit Model"=w44:T30, "NLSF Parameters Map X Resolution"=w50:i32, "NLSF Parameters Map Y Resolution"=w49:i32, "Is Full Image Parameters Map"=w53:bool, "Fit Options: Decay Preprocessing Parameters"=w60:T39, "Fit Options: Reference Decay"=w61:cluster{"t Array":dbl[], "I Array":dbl[]}, "Current Dataset Images 1.SGL Image Sum"=w74:T2, "Current Dataset Images 1.SGL Gate Images"=w73:T2[], "Current Dataset Images 2.SGL Image Sum"=w72:T2, "Current Dataset Images 2.SGL Gate Images"=w71:T2[], "Reference Decay"=w113:cluster{"t Array":dbl[], "I Array":dbl[]}, "[[Multiple Decays Fit Parameters]]"=w91:dbl[][], "IRF Array Time Axis"=w102:dbl[], "[[IRFs]]"=w87:dbl[][], "[Decay Fit Parameter Names]"=w86:T40[], "Decay Fit Options & Parameters"=w83:T28, "[[Multiple Decays Fit Parameter SDVs]]"=w80:dbl[][], "Is Single-Pixels Parameters Map"=w45:bool, "[Decay Sum]"=w41:dbl[], "Selected ROIs Array"=w40:bool[], "[ROI Descriptors]"=w32:T5[])
      n8 = call "AlliGator Get Pixel Count Constraints.vi"("error in (no error)"=w70) -> ("error out"=w120:errorcluster, "Pixel Count Constraints"=w121:T43)  [unwired: 9 in]
      n9 = call "AlliGator Settings Storage.vi"("AlliGator Settings List"=AlliGator_Settings_List."Data Information:Laser Period", "Error In"=w68) -> ("Error Out"=w95:errorcluster, "Variant Data out"=w97:variant)  [unwired: 8 in]
      n10 = call "AlliGator Settings Storage.vi"("AlliGator Settings List"=AlliGator_Settings_List."Fluorescence Decay_Fit Parameters:Export Tabulated Results", "Error In"=w69) -> ("Error Out"=w109:errorcluster, "Variant Data out"=w110:variant)  [unwired: 8 in]
      n11 = call "Alligator Variables Storage.vi"("AlliGator Variable"=AlliGator_Variables_List."Files:Dataset Channel" ("Alligator Variable"), "Error In"=w66) -> ("Error Out"=w65:errorcluster, "Data out"=w63:variant)  [unwired: 7 in, 1 out]
      n12 = call-poly "Variant to Data.vi"("Variant"=w63) -> ("U16 Value"=w62:u16)  [unwired: 8 in]
      n13 = call "AlliGator Get Decay Peak Constraints.vi"("error in (no error)"=w67) -> ("Error Out"=w116:errorcluster, "Decay Peak Constraints"=w115:T46)  [unwired: 9 in]
      n14 = case shown="1" w62 {
        tunnel: [w127 w129] -> w76
        tunnel: w74 -> [w127 _]
        tunnel: [w126 w128] -> w75
        tunnel: w73 -> [w126 _]
        tunnel: w72 -> [_ w129]
        tunnel: w71 -> [_ w128]
        frame 0, Default {
        }
        frame 1 {
        }
      }
      n15 = call-poly "Variant to Data.vi"("Variant"=w110) -> ("Value"=w38:bool)  [unwired: 8 in]
      n16 = call "Alligator Variables Storage.vi"("AlliGator Variable"=AlliGator_Variables_List."Source Image:ROIs" ("Alligator Variable"), "Error In"=w65) -> ("Error Out"=w123:errorcluster, "Data out"=w124:variant)  [unwired: 7 in, 1 out]
      n17 = Variant To Data(error in=w95, type=dbl[unit] 5e-08 ("Laser Period"), Variant=w97) -> (data=w93:dbl[unit], error out=w94:errorcluster)
      n18 = Variant To Data(error in=w123, type=T4[] [] ("Stored ROIs in"), Variant=w124) -> (data=w103:T4[], error out=w119:errorcluster)
      n19 = node(w93) -> (w92:dbl)
      n20 = Bundle By Name(cluster=cluster{"Image Sum":T2, "Image Array":T2[]} {"Image Sum"=refnum, "Image Array"=[]} ("Images"), "Image Sum"=w76, "Image Array"=w75) -> (w114:cluster{"Image Sum":T2, "Image Array":T2[]})
      n21 = call "AlliGator Get Sum Image Threshold.vi"("error in (no error)"=w120, "Pixel Counts Constraints"=w121, "Image in"=w76) -> ("error out"=w85:errorcluster, "Pixel Threshold Low"=w117:sgl, "Pixel Threshold High"=w118:sgl, "Y Resolution"=w56:i32, "X Resolution"=w57:i32)  [unwired: 2 in, 2 out]
      n22 = Array Size(array=w103) -> (size(s)=w55:i32)
      n23 = Multiply(x=w57, y=w56) -> (x*y=w54:i32)
      n24 = Equal?(x=w54, y=w55) -> (x = y?=w51:bool)
      n25 = Merge Errors(w85, w119, w116, w94, w109) -> (w78:errorcluster)
      n26 = case shown="1, Default" w55 {
        selector: w55 -> [_ w193]
        tunnel: w118 -> [_ w236]
        tunnel: w117 -> [_ w235]
        tunnel: w115 -> [_ w234]
        tunnel: w114 -> [_ w233]
        tunnel: w75 -> [_ w232]
        tunnel: w113 -> [_ w184]
        tunnel: [_ w229] -> w112
        tunnel: [_ w226] -> w108
        tunnel: w103 -> [_ w225]
        tunnel: w102 -> [_ w224]
        tunnel: [w143 w223] -> w99
        tunnel: w92 -> [_ w221]
        tunnel: w91 -> [w144 w219]
        tunnel: [w144 w217] -> w90
        tunnel: [_ w152] -> w89
        tunnel: [w145 w216] -> w88
        tunnel: w87 -> [_ w200]
        tunnel: w86 -> [w145 w199]
        tunnel: w78 -> [_ w210]
        tunnel: w38 -> [_ w204]
        tunnel: [w142 w203] -> w84
        tunnel: w83 -> [w142 w189]
        tunnel: [w141 w201] -> w81
        tunnel: w80 -> [w141 w190]
        tunnel: w79 -> [_ w196]
        tunnel: w61 -> [w139 w187]
        tunnel: w60 -> [w138 w188]
        tunnel: [w139 w183] -> w59
        tunnel: [w138 w185] -> w58
        tunnel: w53 -> [w137 w171]
        tunnel: [w137 w177] -> w52
        tunnel: w51 -> [_ w170]
        tunnel: w50 -> [w136 w169]
        tunnel: w49 -> [w135 w173]
        tunnel: [w136 w176] -> w48
        tunnel: [w135 w175] -> w47
        tunnel: [w134 w167] -> w46
        tunnel: w45 -> [w134 w166]
        tunnel: w44 -> [w133 w165]
        tunnel: [w133 w164] -> w43
        tunnel: [w132 w158] -> w42
        tunnel: w41 -> [w132 w157]
        tunnel: w40 -> [w131 w156]
        tunnel: [w131 w155] -> w39
        tunnel: w32 -> [w130 w151]
        tunnel: [w130 w150] -> w31
        frame 0 {
          n27 = One Button Dialog(message="All ROIs Decay Fit: no ROI defined!") -> ()  [unwired: 1 in, 1 out]
          n28 = call "Play Error Sound.vi"() -> ()  [unwired: 27 in, 1 out]
          n29 = xnode "Error Ring"() -> ("error out"=w143:errorcluster)
        }
        frame 1, Default {
          # "the second pass idea requires another way to pass best fit parameters to // loops: now inactive"
          # "invalid fit [idx]\noriginally: all"
          n30 = call "AlliGator Get-Set Decay Preprocessing Parameters.vi"("Get (F)/Set"=FALSE, "Error In"=w210) -> ("Error Out"=w182:errorcluster, "Decay Preprocessing Parameters out"=w186:T39)  [unwired: 8 in]
          n31 = call "AlliGator Get Fit Options & Parameters.vi"("error in (no error)"=w182, "Reset Fit Options & Parameters"=TRUE) -> ("error out"=w181:errorcluster, "Use Legacy Fitting Approach"=w180:bool, "Decay Fit Options & Parameters"=w178:T28)  [unwired: 7 in]
          n32 = call "AlliGator New NLSF Parameter Map Resolution.vi"("Is Full Image Parameter Map"=w170, "Old NLSF Parameters Map Y Resolution"=w173, "Old NLSF Parameters Map X Resolution"=w169) -> (2:"New NLSF Parameters Map X Resolution"=w172:i32, 3:"New NLSF Parameters Map X Resolution"=w174:i32)  [unwired: 7 in]
          n33 = Array Size(array=w232) -> (size(s)=w231:i32)
          n34 = call "AlliGator Get IRF Values & Locations.vi"("[IRF Data]"=w200) -> ("IRF Locations"=w160:cluster{"X":i32, "Y":i32}[], "[IRF Values]"=w161:dbl[][])  [unwired: 9 in]
          n35 = call "Embedded Progress Bar Q.vi"("Progress Bar Queue Name"="AlliGator Progress Bar Q") -> ("Progress Bar Queue"=w195:refnum<queue>)  [unwired: 6 in]
          n36 = call "Linear Ramp [I32].vi"("# Elements"=w193) -> ("Ramp"=w209:i32[])  [unwired: 8 in]
          n37 = call "AlliGator Get Decay Time Axis v2.vi"("Number of Gates"=w231) -> ("t Array"=w230:dbl[unit][])  [unwired: 14 in]
          n38 = call "Send Embedded Progress Bar Update.vi"("Max Iterations N"=w193, "Current Iteration i (i or -1: standard or || iteration; 0 or -2: first standard or || iteration)"=-2 ("Current Iteration i (i or -1: standard or || iteration; 0 or -2: first standard or || iteration)"), "Progress Bar Queue in"=w195) -> ("Error Out"=w191:errorcluster, "Progress Bar Queue out"=w194:refnum<queue>)  [unwired: 7 in]
          n39 = call "Logical Processors Used.vi"() -> ("# Logical Processor Used"=w162:i32)  [unwired: 6 in]
          n40 = node(w230) -> (w228:dbl[])
          n41 = for {
            N: 1 -> [_]
            tunnel: w236 -> [w293]
            tunnel: w235 -> [w292]
            tunnel: w234 -> [w291]
            tunnel: w233 -> [w290]
            tunnel: w184 -> [w289]
            tunnel: [w249] -> w229 mode=concatenating
            tunnel: w228 -> [w288]
            tunnel: "Abort Fit" ("Abort Button Name (Abort)") -> [w287]
            tunnel: [w286] -> w226
            tunnel: w224 -> [w284]
            tunnel: w197 -> [w281]
            tunnel: [w279] -> w222 mode=concatenating
            tunnel: w221 -> [w278]
            shift-right: [w273] -> w152
            shift-left: _ -> [w276]
            tunnel: w204 -> [w282]
            tunnel: [FALSE ("Abort?")] -> w220
            shift-right: [w274] -> _
            shift-left: dbl[][] [] -> [w264]
            tunnel: [w277] -> w218 mode=concatenating
            tunnel: [w271] -> w214
            tunnel: w181 -> [w269]
            tunnel: w161 -> [w283]
            shift-right: [w268] -> _
            shift-left: i32[] [] -> [w263]
            tunnel: w225 -> [w285]
            tunnel: w193 -> [w280]
            shift-right: [w267] -> _
            shift-left: w209 -> [w255]
            tunnel: [w262] -> w202 mode=concatenating
            tunnel: w160 -> [w261]
            tunnel: w186 -> [w260]
            tunnel: w196 -> [w256]
            tunnel: w194 -> [w265]
            tunnel: [w270] -> w213
            tunnel: w191 -> [w253]
            tunnel: w178 -> [w252]
            tunnel: w180 -> [w251]
            tunnel: [w246] -> w168
            tunnel: [w245] -> w163
            tunnel: w162 -> [w244]
            tunnel: [w243] -> w159 mode=concatenating
            tunnel: [w242] -> w154 mode=concatenating
            tunnel: [w241] -> w153 mode=concatenating
            i -> [w259]
            stop <- w272 stop-if-true
            # "invalid fit idx\n(unused)"
            # "First Loop: try all decays [deprecated: Second Loop: try all the failed decay fit again with parameters from nearby successful fits]"
            n42 = Array Size(array=w255) -> (size(s)=w254:i32)
            n43 = for {
              tunnel: w285 -> [w324] mode=indexing
              tunnel: w293 -> [w344]
              tunnel: w292 -> [w343]
              tunnel: w290 -> [w342]
              tunnel: w291 -> [w341]
              tunnel: w288 -> [w340]
              tunnel: w289 -> [w339]
              tunnel: [w338] -> w249 mode=indexing if=w332
              tunnel: w269 -> [w322]
              tunnel: w287 -> [w337]
              tunnel: [w336] -> w279 mode=indexing if=w300
              tunnel: [w335] -> w286 mode=indexing if=w300
              tunnel: w282 -> [w333]
              tunnel: [w334] -> w277 mode=indexing if=w300
              tunnel: w280 -> [w319]
              tunnel: w284 -> [w331]
              tunnel: w283 -> [w323]
              tunnel: [w308] -> w273
              tunnel: w281 -> [w330]
              tunnel: [w328] -> w271
              tunnel: w278 -> [w326]
              tunnel: w276 -> [w325]
              tunnel: [w316] -> w267 mode=indexing if=w318
              tunnel: w255 -> [w321]
              tunnel: [w313] -> w262 mode=indexing if=w300
              tunnel: w261 -> [w312]
              tunnel: w260 -> [w311]
              tunnel: w265 -> [w329]
              tunnel: [w327] -> w270
              tunnel: w253 -> [w310]
              tunnel: w264 -> [w314]
              tunnel: [w317] -> w274 mode=indexing if=w300
              tunnel: w263 -> [w315]
              tunnel: [w316] -> w268 mode=indexing if=w300
              tunnel: w252 -> [w307]
              tunnel: w251 -> [w306]
              tunnel: [w305] -> w250 mode=indexing if=w300
              tunnel: [w304] -> w245
              workers-P: w244 -> [_]
              tunnel: [w303] -> w243 mode=indexing if=w300
              tunnel: [TRUE ("Abort?")] -> w242 mode=indexing if=w300
              tunnel: [w301] -> w241 mode=indexing if=w300
              i -> [w320]
              n44 = global read "AlliGator Abort.vi" "Abort?"() -> (w308:bool)
              n45 = case shown="False" w308 {
                selector: w308 -> [w351 _]
                tunnel: w344 -> [w383 _]
                tunnel: w343 -> [w382 _]
                tunnel: w342 -> [w381 _]
                tunnel: w341 -> [w380 _]
                tunnel: w340 -> [w379 _]
                tunnel: w339 -> [w378 _]
                tunnel: [w377 _] -> w338
                tunnel: w337 -> [w376 _]
                tunnel: [w375 w476] -> w336
                tunnel: [w374 _] -> w335
                tunnel: [w373 _] -> w334
                tunnel: w333 -> [w372 _]
                tunnel: [w371 _] -> w332
                tunnel: w331 -> [w370 _]
                tunnel: w330 -> [w369 _]
                tunnel: w326 -> [w368 _]
                tunnel: w325 -> [_ _]
                tunnel: w324 -> [w367 _]
                tunnel: w323 -> [w366 _]
                tunnel: w322 -> [w365 w476]
                tunnel: w321 -> [w364 _]
                tunnel: w320 -> [w362 _]
                tunnel: w319 -> [w361 _]
                tunnel: [w360 _] -> w318
                tunnel: [w359 _] -> w317
                tunnel: [w358 _] -> w316
                tunnel: w315 -> [w357 _]
                tunnel: w314 -> [w356 _]
                tunnel: [w355 _] -> w313
                tunnel: w312 -> [w354 _]
                tunnel: w311 -> [w353 _]
                tunnel: [w352 _] -> w300
                tunnel: w307 -> [w350 _]
                tunnel: w306 -> [w349 _]
                tunnel: [w348 _] -> w305
                tunnel: [w347 _] -> w304
                tunnel: [w346 _] -> w303
                tunnel: [w345 _] -> w301
                frame False {
                  n46 = Search 1D Array(1D array=w364, element=w362) -> (index of element=w363:i32)  [unwired: 1 in]
                  n47 = case shown="0, Default" w363 {
                    tunnel: w383 -> [w430 _]
                    tunnel: w382 -> [w429 _]
                    tunnel: w381 -> [w428 _]
                    tunnel: w380 -> [w427 _]
                    tunnel: w379 -> [w426 _]
                    tunnel: w378 -> [w422 _]
                    tunnel: [w421 _] -> w377
                    tunnel: w376 -> [w420 _]
                    tunnel: [w419 _] -> w375
                    tunnel: [w418 _] -> w374
                    tunnel: [w417 _] -> w373
                    tunnel: w372 -> [w416 _]
                    tunnel: [w415 _] -> w371
                    tunnel: w370 -> [w414 _]
                    tunnel: w369 -> [w410 _]
                    tunnel: w361 -> [w409 _]
                    tunnel: w368 -> [w408 _]
                    tunnel: w367 -> [w407 _]
                    tunnel: w366 -> [w397 _]
                    tunnel: [w406 _] -> w359
                    tunnel: w362 -> [w386 _]
                    tunnel: w365 -> [w402 _]
                    tunnel: [w405 _] -> w358
                    tunnel: [w403 _] -> w352
                    tunnel: [w404 _] -> w360
                    tunnel: w357 -> [_ _]
                    tunnel: w356 -> [_ _]
                    tunnel: w362 -> [_ _]
                    tunnel: [w400 _] -> w355
                    tunnel: w354 -> [w399 _]
                    tunnel: w353 -> [w394 _]
                    tunnel: w351 -> [w393 _]
                    tunnel: w350 -> [w391 _]
                    tunnel: w349 -> [w390 _]
                    tunnel: [w388 _] -> w348
                    tunnel: [w387 _] -> w347
                    tunnel: [w385 _] -> w346
                    tunnel: [w384 _] -> w345
                    frame 0, Default {
                      # "corresponding IRF location found?"
                      n48 = Unbundle By Name(w407) -> ("ROI Descriptor"=w384:T5, "ROI Name"=w421:string)
                      n49 = call "AlliGator Compute ROI Decay.vi"("Pixel Threshold High"=w430, "Loop ID"=w386, "Pixel Threshold Low"=w429, "error in (no error)"=w402, "Decay Peak  Constraints"=w427, "ROI Descriptor"=w384, "Images"=w428) -> ("error out"=w401:errorcluster, "# Valid Pixels"=w423:i32, "ROI Center"=w398:cluster{"X":i32, "Y":i32}, "Decay Points"=w425:dbl[], "# Pixels"=w389:i32)
                      n50 = To Double Precision Float(number=w398) -> (double precision float=w413:cluster{"X":dbl, "Y":dbl})
                      n51 = Search 1D Array(1D array=w399, element=w398) -> (index of element=w395:i32)  [unwired: 1 in]
                      n52 = Cluster To Array(cluster=w413) -> (array=w412:dbl[])
                      n53 = Index Array(array=w397, index (row)=w395) -> (element=w396:dbl[])  [unwired: 1 in]
                      n54 = Greater Or Equal To 0?(x=w395) -> (x >= 0?=w392:bool)
                      n55 = Bundle(w426, "Decay Points"=w425) -> (w424:cluster{dbl[], "Decay Points":dbl[]})  [unwired: 1 in]
                      n56 = Compound Arithmetic op=AND(w392, invert w393) -> (w411:bool)
                      n57 = case shown="True" w411 {
                        tunnel: w424 -> [_ w472]
                        tunnel: w423 -> [_ w471]
                        tunnel: w422 -> [_ w470]
                        tunnel: w421 -> [_ w468]
                        tunnel: w420 -> [_ _]
                        tunnel: [w431 w452] -> w419
                        tunnel: [_ w466] -> w418
                        tunnel: [_ w455] -> w417
                        tunnel: w416 -> [_ w464]
                        tunnel: w409 -> [_ w463]
                        tunnel: w386 -> [_ w448]
                        tunnel: [_ w462] -> w415
                        tunnel: w414 -> [_ w460]
                        tunnel: w412 -> [_ w437]
                        tunnel: w401 -> [w431 w458]
                        tunnel: w410 -> [_ w446]
                        tunnel: w408 -> [_ w445]
                        tunnel: [_ w453] -> w406
                        tunnel: [_ w448] -> w405
                        tunnel: [_ TRUE] -> w403
                        tunnel: [_ w443] -> w400
                        tunnel: w396 -> [_ w442]
                        tunnel: w394 -> [_ w441]
                        tunnel: w391 -> [_ w436]
                        tunnel: w390 -> [_ w440]
                        tunnel: w389 -> [_ w438]
                        tunnel: [_ w438] -> w388
                        tunnel: [_ w435] -> w387
                        tunnel: [_ w432] -> w385
                        frame False {
                          # "Not the same ROI coordinates"
                        }
                        frame True {
                          w469 = T47 {"Multiplot XY Graph"=refnum, "Mouse Coordinates"={"Horizontal"=0, "Vertical"=0}, "Plot Index"=-1, "Flag"=FALSE}  # Flag: non-interactive
                          n58 = call "AlliGator Preprocess Decay v3.vi"("Decay Preprocessing Parameters"=w441, "Error In"=w458, "Time-Gated Reference Decay"=w470, "# Pixels"=w471, "Decay (in)"=w472) -> ("Error Out"=w454:errorcluster, "Decay (out)"=w434:T50)  [unwired: 3 in, 2 out]
                          n59 = Bundle("IRF Array Time Axis"=w460, "[IRF Values]"=w442) -> (w459:T51)  [unwired: 1 in]
                          n60 = call "AlliGator Fit Decay.vi"("Selected Plot Info + Flag"=w469, "Decay Fit Options & Parameters"=w436, "Current Decay Name"=w468, "Current Decay"=w434, "Reference Decay"=w459, "error in (no error)"=w454, "Use Legacy Fitting Approach"=w440) -> ("Best Fit Parameters (All)"=w453:dbl[], "Delta Best Fit Parameters (All)"=w447:dbl[], "R^2"=w439:dbl, "Reduced Chi^2"=w467:dbl, "Error Out"=w452:errorcluster)  [unwired: 4 out]
                          n61 = Unbundle By Name(w434) -> ("ROI Intensity Array"=w433:dbl[])
                          n62 = Unbundle By Name(w452) -> ("status"=w451:bool)
                          n63 = call "Keep String in Array.vi"("Current Index"=w448, "Number of Elements"=w463) -> ("Keep String"=w461:bool)  [unwired: 9 in]
                          n64 = Build Array (concatenate)(w453, w439, w467) -> (w457:dbl[])
                          n65 = Not(x=w451) -> (.not. x?=w450:bool)
                          n66 = call "Get Decay Fit Parameters.vi"("Laser Period"=w445, "Decay Fit Output Options"=w446, "Decay Fit Parameters"=w457) -> ("Displayed Decay Fits Parameters"=w456:dbl[])  [unwired: 7 in, 1 out]
                          n67 = Build Array (concatenate)(w437, w457) -> (w465:dbl[])
                          n68 = Unbundle By Name(w436) -> ("Fit Options.Fit Model"=w435:T30)
                          n69 = Add Array Elements(numeric array=w433) -> (sum=w432:dbl)
                          n70 = call "Get Decay Fit Parameters.vi"("Laser Period"=w445, "Decay Fit Output Options"=w446, "Decay Fit Parameters"=w447) -> ("Displayed Decay Fits Parameters"=w444:dbl[])  [unwired: 7 in, 1 out]
                          n71 = case shown="True" w464 {
                            tunnel: [_ w475] -> w466
                            tunnel: w465 -> [_ w474]
                            frame False {
                            }
                            frame True {
                              n72 = Array To Spreadsheet String(array=w474, 3:"%#g" ("format string")) -> (spreadsheet string=w475:string)  [unwired: 1 in]
                            }
                          }
                          n73 = Build Array (concatenate)(w437, w456) -> (w455:dbl[])
                          n74 = Build Array (concatenate)(w437, w444) -> (w443:dbl[])
                          n75 = Compound Arithmetic op=AND(w461, w450) -> (w462:bool)
                        }
                      }
                      n76 = Not(x=w403) -> (.not. x?=w404:bool)
                    }
                    frame -1 {
                      # "already successful: do nothing"
                    }
                  }
                }
                frame True {
                }
              }
              n77 = call "Send Embedded Progress Bar Update.vi"("Error In"=w310, "Current Iteration i (i or -1: standard or || iteration; 0 or -2: first standard or || iteration)"=-1 ("Current Iteration i (i or -1: standard or || iteration; 0 or -2: first standard or || iteration)"), "Progress Bar Queue in"=w329) -> ("Error Out"=w328:errorcluster, "Progress Bar Queue out"=w327:refnum<queue>)  [unwired: 7 in]
            }
            n78 = case shown="0, Default" w259 {
              tunnel: [w295 w299] -> w257
              tunnel: w254 -> [_ w297]
              frame 0, Default {
                n79 = call "Current Date & Time String (High Precision).vi"() -> ("on <Date> at <Time>"=w294:string)  [unwired: 8 in, 3 out]
                n80 = Format Into String(format string="All ROIs Non-Interactive Decay Fit (Individual IRFs) started %s", w294) -> (resulting string=w295:string)  [unwired: 2 in, 1 out]
              }
              frame 1 {
                n81 = Format Into String(format string="Re-processing %d decays...", w297) -> (resulting string=w299:string)  [unwired: 2 in, 1 out]
              }
            }
            n82 = call "Get Current Message Text Format.vi"("Text Format"=Text_Format_List."Result") -> ("Message Formatting"=w258:T52)  [unwired: 8 in, 1 out]
            n83 = call "Send Message to Notebook.vi"("Text Formatting"=w258, "Text"=w257, "Notebook Queue"=w256) -> ()  [unwired: 5 in, 2 out]
            n84 = Empty Array?(array=w267) -> (empty?=w266:bool)
            n85 = Add Array Elements(numeric array=w250) -> (sum=w247:i32)
            n86 = Array Size(array=w249) -> (size(s)=w248:i32)
            n87 = Equal?(x=w248, y=w247) -> (x = y?=w246:bool)
            n88 = Compound Arithmetic op=OR(w266, w273) -> (w272:bool)
          }
          n89 = flat-sequence {
            tunnel: [w238] -> w205
            tunnel: [w237] -> w197
            frame #0 {
              n90 = call "AlliGator Get Fit Output Options.vi"("All Parameters?"=TRUE) -> ("Decay Fit Output Options"=w237:T56)  [unwired: 8 in, 2 out]
              n91 = Unbundle By Name(w237) -> ("Decay Fit Parameter Array"=w238:T40[])
            }
          }
          n92 = global write "AlliGator Abort.vi" "Abort?"(w220) -> ()
          n93 = call "Send Embedded Progress Bar Update.vi"("Stop Progress Bar (F)"=TRUE ("Hide Progress Bar"), "Error In"=w214, "Progress Bar Queue in"=w213) -> ("Error Out"=w212:errorcluster)  [unwired: 7 in, 1 out]
          n94 = Select(t=w187, s=w152, f=w184) -> (s? t:f=w183:cluster{"t Array":dbl[], "I Array":dbl[]})
          n95 = Select(t=w190, s=w152, f=w202) -> (s? t:f=w201:dbl[][])
          n96 = Select(t=w219, s=w152, f=w218) -> (s? t:f=w217:dbl[][])
          n97 = Select(t=w199, s=w152, f=w205) -> (s? t:f=w216:T40[])
          n98 = Select(t=w188, s=w152, f=w186) -> (s? t:f=w185:T39)
          n99 = Merge Errors(w222, w212) -> (w223:errorcluster)
          n100 = Select(t=w171, s=w152, f=w170) -> (s? t:f=w177:bool)
          n101 = Select(t=w189, s=w152, f=w178) -> (s? t:f=w203:T28)
          n102 = Select(t=w157, s=w152, f=w159) -> (s? t:f=w158:dbl[])
          n103 = Select(t=w173, s=w152, f=w172) -> (s? t:f=w175:i32)
          n104 = Select(t=w156, s=w152, f=w154) -> (s? t:f=w155:bool[])
          n105 = Select(t=w151, s=w152, f=w153) -> (s? t:f=w150:T5[])
          n106 = Select(t=w166, s=w152, f=w168) -> (s? t:f=w167:bool)
          n107 = Select(t=w169, s=w152, f=w174) -> (s? t:f=w176:i32)
          n108 = Select(t=w165, s=w152, f=w163) -> (s? t:f=w164:T30)
        }
      }
      n109 = call "AlliGator Get Tabulated Results Header (Decay Fit).vi"() -> ("Tabulated Results Header"=w107:string)  [unwired: 10 in, 1 out]
      n110 = call <vilib>:"Clear Errors.vi"("error in (no error)"=w99, "specific error code to clear (0: all)"=w82) -> ("error out"=w37:errorcluster)  [unwired: 4 in, 1 out]
      n111 = call "Alligator Variables Storage.vi"("Get(F)/Set"=TRUE, "AlliGator Variable"=AlliGator_Variables_List."Decay Fit Parameter Map:Decay Fit Result Constraints Applied" ("Alligator Variable"), "Error In"=w37, "Data in"=FALSE) -> ("Error Out"=w36:errorcluster)  [unwired: 5 in, 2 out]
      n112 = Build Array (concatenate)(w107, w108) -> (w106:string[])
      n113 = in-place-cluster #2("Fit Model"=w43, "NLSF Parameters Map X Resolution"=w48, "NLSF Parameters Map Y Resolution"=w47, "Is Full Image Parameters Map"=w52, "Fit Options: Decay Preprocessing Parameters"=w58, "Fit Options: Reference Decay"=w59, "Current Dataset Images 1.SGL Image Sum"=w74, "Current Dataset Images 1.SGL Gate Images"=w73, "Current Dataset Images 2.SGL Image Sum"=w72, "Current Dataset Images 2.SGL Gate Images"=w71, "Reference Decay"=w113, "[[Multiple Decays Fit Parameters]]"=w90, "IRF Array Time Axis"=w102, "[[IRFs]]"=w87, "[Decay Fit Parameter Names]"=w88, "Decay Fit Options & Parameters"=w84, "[[Multiple Decays Fit Parameter SDVs]]"=w81, "Is Single-Pixels Parameters Map"=w46, "[Decay Sum]"=w42, "Selected ROIs Array"=w39, "[ROI Descriptors]"=w31) -> (w29:T7)
      n114 = case shown="False" w89 {
        tunnel: w106 -> [w483 _]
        tunnel: [w482 w496] -> w105
        tunnel: w36 -> [w481 w496]
        tunnel: "Choose or enter file path for tabulated fits results:" ("prompt (Choose or enter file path)") -> [w480 _]
        tunnel: "Fit Results saved in %s" ("format string") -> [w479 _]
        tunnel: [w478 "All ROIs Decay Fit (Non-interactive, Individual IRF) aborted by user."] -> w100
        tunnel: w38 -> [w477 _]
        frame False {
          # "Don't Abort"
          n115 = case shown="True" w477 {
            tunnel: w483 -> [_ w494]
            tunnel: [w484 w487] -> w482
            tunnel: w481 -> [w484 w493]
            tunnel: w480 -> [_ w492]
            tunnel: w479 -> [_ w486]
            tunnel: [_ w485] -> w478
            frame False {
            }
            frame True {
              n116 = Write to Text File(prompt (Choose or enter file path)=w492, text=w494, error in=w493) -> (refnum out=w491:refnum<file>, error out=w490:errorcluster)  [unwired: 1 in, 1 out]
              n117 = Close File(refnum=w491, error in=w490) -> (path=w488:path, error out=w489:errorcluster)
              n118 = Format Into String(format string=w486, error in=w489, w488) -> (resulting string=w485:string, error out=w487:errorcluster)  [unwired: 1 in]
            }
          }
        }
        frame True {
          # "Abort"
        }
      }
    }
    n119 = in-place-dvr #1(w29) -> (→"AlliGator Internal Variables DVR":refnum<data-value>)  [unwired: 1 out]
  }
  n120 = call "High Resolution Timing.vi"("relative seconds (NaN)"=w14, "Error In"=w9) -> ("elapsed (relative) seconds"=w13:dbl, "Error Out"=w7:errorcluster)  [unwired: 15 in, 1 out]
  n121 = call "Concatenate String Array.vi"("Max Number of Elements (None: -1)"=8 ("Max Number of Elements (None: 1)"), "Separator (TAB)"=", ", "String Array"=w11) -> ("Formatted String"=w12:string)  [unwired: 8 in]
  n122 = call "Current Date & Time String (High Precision).vi"("Error In"=w7) -> ("Error Out"=w6:errorcluster, "on <Date> at <Time>"=w1:string)  [unwired: 7 in, 2 out]
  n123 = Format Into String(format string="All ROIs Decay Fit (%d):\n%s completed on %s\nCPU: %#g s\n%s", error in=w6, w5, w12, w1, w13, w8) -> (resulting string=→"Message":string, error out=→"error out":errorcluster)  [unwired: 1 in]
